vi "Configure USB Trigger Source.vi"(0 "VISA resource name":refnum<visa-resource-name>, 1 "D+ (0: Channel 1)":u16(ring) items=["Channel 1", "Channel 2", "Channel 3", "Channel 4", "DIG 0", "DIG 1", "DIG 2", "DIG 3", "DIG 4", "DIG 5", "DIG 6", "DIG 7", "DIG 8", "DIG 9", "DIG 10", "DIG 11", "DIG 12", "DIG 13", "DIG 14", "DIG 15", "External"], 5 "Trigger (0: Start of Packet)":u16(ring) items=["Start of Packet", "End of packet", "Reset complete", "Enter suspend state", "Exit suspend state"], 9 "Speed (1: Full Speed)":u16(ring)=1 items=["Low Speed", "Full Speed"], 11 "error in (no error)":errorcluster, 12 "D-  (1: Channel 2)":u16(ring)=1 items=["Channel 1", "Channel 2", "Channel 3", "Channel 4", "DIG 0", "DIG 1", "DIG 2", "DIG 3", "DIG 4", "DIG 5", "DIG 6", "DIG 7", "DIG 8", "DIG 9", "DIG 10", "DIG 11", "DIG 12", "DIG 13", "DIG 14", "DIG 15", "External"]) -> (4 "VISA resource name out":refnum<visa-resource-name>, 15 "error out":errorcluster)   [LabVIEW 2017, in "Agilent 6000 Series.lvlib"]
doc: "This VI configures the USB trigger. You specify the trigger, speed, D+ and D- with the Trigger, Speed, D+ and D- parameters.\n\n<B>NOTE:</B>\n\nThis VI is only valid for 6000 Series models. An error will be thrown if this VI is run with 5000 Series scopes."
uses:
  <instrlib>/Agilent 6000 Series/Agilent 6000 Series.lvlib
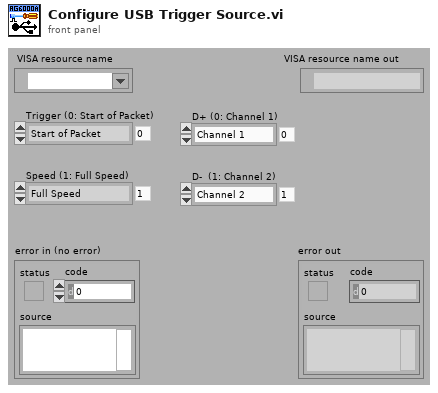
[diagram p1: front panel]
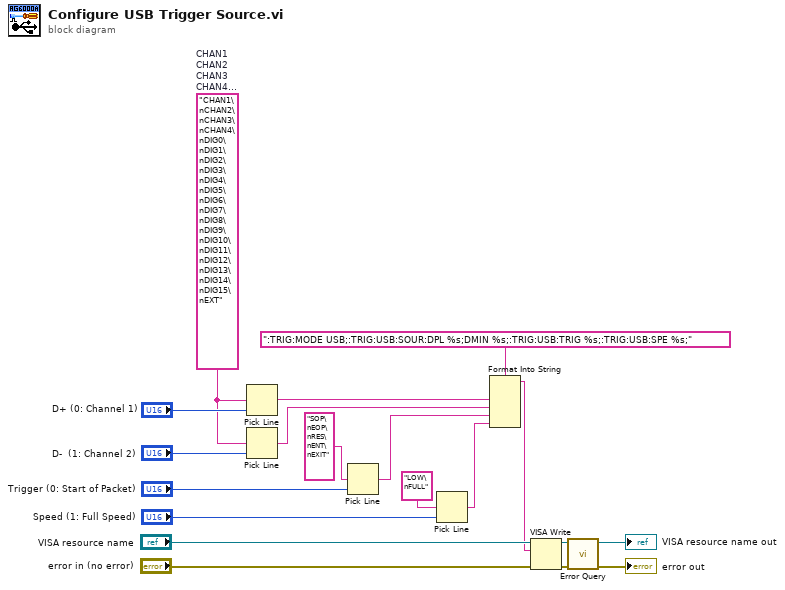
[diagram p0: block diagram]
diagram:
  w8 = "CHAN1\nCHAN2\nCHAN3\nCHAN4\nDIG0\nDIG1\nDIG2\nDIG3\nDIG4\nDIG5\nDIG6\nDIG7\nDIG8\nDIG9\nDIG10\nDIG11\nDIG12\nDIG13\nDIG14\nDIG15\nEXT"  # CHAN1 CHAN2 CHAN3 CHAN4 DIG0 DIG1 DIG2 DIG3 DIG4 DIG5 DIG6 DIG7 DIG8 DIG9 DIG10 DIG11 DIG12 DIG13 DIG14 DIG15 EXT
  n1 = Pick Line(multi-line string=w8, line index="D+ (0: Channel 1)") -> (output string=w12:string)  [unwired: 1 in]
  n2 = Pick Line(multi-line string=w8, line index="D-  (1: Channel 2)") -> (output string=w7:string)  [unwired: 1 in]
  n3 = Pick Line(multi-line string="SOP\nEOP\nRES\nENT\nEXIT", line index="Trigger (0: Start of Packet)") -> (output string=w4:string)  [unwired: 1 in]
  n4 = Pick Line(multi-line string="LOW\nFULL", line index="Speed (1: Full Speed)") -> (output string=w1:string)  [unwired: 1 in]
  n5 = Format Into String(format string=":TRIG:MODE USB;:TRIG:USB:SOUR:DPL %s;DMIN %s;:TRIG:USB:TRIG %s;:TRIG:USB:SPE %s;" ("Source Command"), w12, w7, w4, w1) -> (resulting string=w10:string)  [unwired: 2 in, 1 out]
  n6 = VISA Write(VISA resource name="VISA resource name", write buffer=w10, error in (no error)="error in (no error)") -> (VISA resource name out=w15:refnum<visa-resource-name>, error out=w14:errorcluster)  [unwired: 1 out]
  n7 = call <instrlib>:"Error Query.vi"("error in (no error)"=w14, "VISA resource name"=w15) -> ("error out"=→"error out":errorcluster, "VISA resource name out"=→"VISA resource name out":refnum<visa-resource-name>)  [unwired: 6 in, 2 out]
